vi "Set Robot Position.vi"(7 "robot position":T1={"global x"=0.0, "global y"=0.0, "global theta"=0.0, "ccw wheel angles"=[0.0, 0.0, 0.0]}, 8 "error in (no error)":errorcluster, 9 "axles":refnum<vi>[](array[refnum]), 10 "robot":refnum<vi>, 11 "scene":refnum<vi>) -> (0 "error out":errorcluster, 3 "scene out":refnum<vi>)   [LabVIEW 2015]
doc: "Reads the position data of the robot, and updates the 3D drawing.s"
uses:
  Robot Position.ctl
  <vilib>/picture/3D Picture Control/NI_3D Picture Control.lvlib
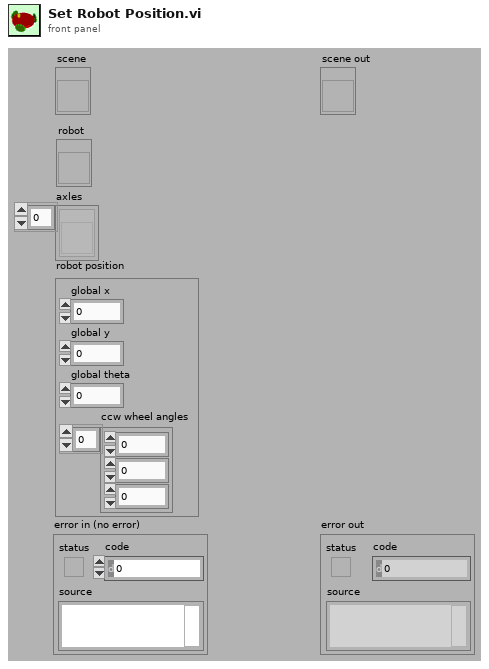
[diagram p1: front panel]
types:
  T1 = typedef "Robot Position.ctl" = cluster{"global x":dbl, "global y":dbl, "global theta":dbl, "ccw wheel angles":dbl[]}
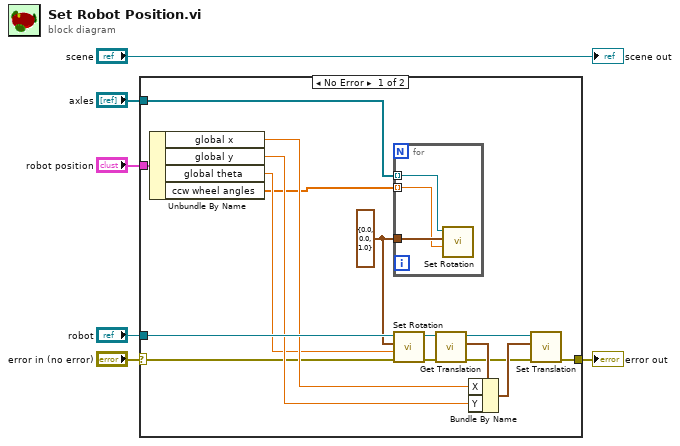
[diagram p0: block diagram]
diagram:
  n1 = case shown="No Error" "error in (no error)" {
    selector: "error in (no error)" -> [w7 w26]
    tunnel: "axles" -> [w22 _]
    tunnel: "robot" -> [w21 _]
    tunnel: "robot position" -> [w19 _]
    tunnel: [w8 w26] -> w2
    frame No Error {
      w20 = cluster{"X":sgl, "Y":sgl, "Z":sgl} {"X"=0.0, "Y"=0.0, "Z"=1.0} ("Axis")
      n2 = Unbundle By Name(w19) -> ("global x"=w18:dbl, "global y"=w17:dbl, "global theta"=w16:dbl, "ccw wheel angles"=w15:dbl[])
      n3 = for {
        tunnel: w22 -> [w24] mode=indexing
        tunnel: w20 -> [w25]
        tunnel: w15 -> [w23] mode=indexing
        n4 = call <vilib>:"Set Rotation.vi"("Angle"=w23, "Axis"=w25, "Scene Object"=w24) -> ()  [unwired: 1 in, 8 out]
      }
      n5 = call <vilib>:"Set Rotation.vi"("error in (no error)"=w7, "Angle"=w16, "Axis"=w20, "Scene Object"=w21) -> ("error out"=w12:errorcluster, "Rotated Scene Object"=w14:refnum<vi>)  [unwired: 6 out]
      n6 = call <vilib>:"Get Translation.vi"("error in (no error)"=w12, "Scene Object"=w14) -> ("error out"=w9:errorcluster, "Transformation:Get Translation"=w11:cluster{"X":sgl, "Y":sgl, "Z":sgl}, "Scene Object"=w13:refnum<vi>)  [unwired: 7 in]
      n7 = Bundle By Name(cluster=w11, "X"=w18, "Y"=w17) -> (w10:cluster{"X":sgl, "Y":sgl, "Z":sgl})
      n8 = call <vilib>:"Set Translation.vi"("error in (no error)"=w9, "Translation"=w10, "Scene Object"=w13) -> ("error out"=w8:errorcluster)  [unwired: 8 out]
    }
    frame Error {
    }
  }
  "error out" <- w2
  "scene out" <- "scene"
